vi "Update Pin Map.vi"(8 "error in":errorcluster, 11 "Pin Map Path":string) -> (0 "error out":errorcluster, 3 "Pin Map Id Out":string)   [LabVIEW 2020, in "NIDCPowerSourceDCVoltage.lvlib"]
uses:
  NIDCPowerSourceDCVoltage.lvlib
  <vilib>/MeasurementLink/MeasurementLink Discovery Client/RPC Messages/ni_measurementlink_discovery_v1_ResolveServiceRequest.ctl
  <vilib>/MeasurementLink/MeasurementLink Pin Map Client/RPC Messages/ni_measurementlink_pinmap_v1_UpdatePinMapFromXmlRequest.ctl
  <vilib>/MeasurementLink/MeasurementLink Measurement Server/MeasurementLink Measurement Server.lvlib
  <vilib>/MeasurementLink/MeasurementLink Discovery Client/MeasurementLink Discovery Client.lvlib
  <vilib>/MeasurementLink/MeasurementLink Pin Map Client/MeasurementLink Pin Map Client.lvlib
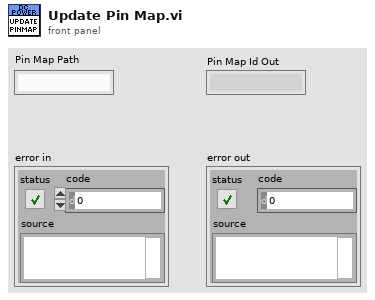
[diagram p1: front panel]
types:
  T1 = typedef "MeasurementLink Pin Map Client.lvlib/ni_measurementlink_pinmap_v1_UpdatePinMapFromXmlRequest.ctl" = cluster{"pin_map_id":string, "pin_map_xml":string}
  T2 = typedef "MeasurementLink Discovery Client.lvlib/ni_measurementlink_discovery_v1_ResolveServiceRequest.ctl" = cluster{"provided_interface":string, "service_class":string}
  T3 = typedef "grpc-lvsupport-release.lvlib/grpcId.ctl" = u64
  T4 = typedef "MeasurementLink Discovery Client.lvlib/ni_measurementlink_discovery_v1_ServiceLocation.ctl" = cluster{"location":string, "insecure_port":string, "ssl_authenticated_port":string}
  T5 = typedef "MeasurementLink Pin Map Client.lvlib/ni_measurementlink_pinmap_v1_PinMap.ctl" = cluster{"pin_map_id":string}
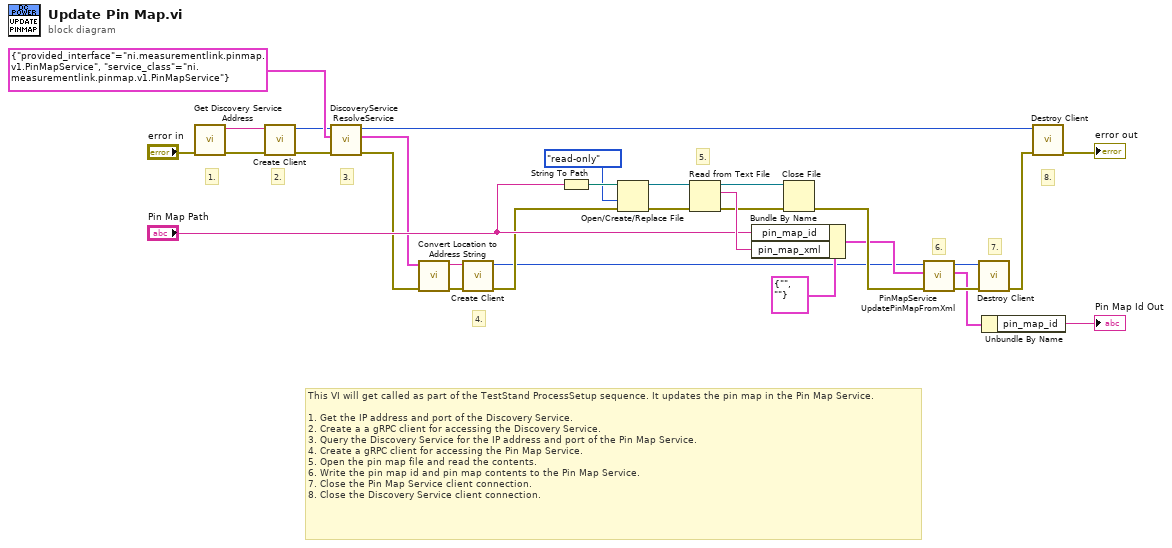
[diagram p0: block diagram]
diagram:
  # "8."
  # "7."
  # "6."
  # "5."
  # "4."
  # "3."
  # "2."
  # "1."
  # "This VI will get called as part of the TestStand ProcessSetup sequence. It updates the pin map in the Pin Map Service. \n\n1. Get the IP address and port of the Discovery Service.\n2. Create a a gRPC client for accessing the Discovery Service.\n3. Query the Discovery Service for the IP address and port of the Pin Map Service.\n4. Create a gRPC client for accessing the Pin Map Service.\n5. Open the pin map file and read the contents.\n6. Write the pin map id and pin map contents to the Pin Map Service.\n7. Close the Pin Map Service client connection.\n8. Close the Discovery Service client connection."
  n1 = call <vilib>:"Get Discovery Service Address.vi"("error in"="error in") -> ("error out"=w29:errorcluster, "address"=w28:string)  [unwired: 9 in]
  n2 = call <vilib>:"Create Client.vi"("error in"=w29, "address"=w28) -> ("error out"=w16:errorcluster, "gRPC ID Out"=w26:T3)  [unwired: 8 in]
  n3 = call <vilib>:"DiscoveryService ResolveService.vi"("error in"=w16, "Request Data"=T2 {"provided_interface"="ni.measurementlink.pinmap.v1.PinMapService", "service_class"="ni.measurementlink.pinmap.v1.PinMapService"}, "gRPC ID"=w26) -> ("error out"=w15:errorcluster, "Response Data"=w4:T4, "gRPC ID out"=w5:T3)  [unwired: 6 in]
  n4 = call "Convert Location to Address String.vi"("Response Data"=w4) -> ("String"=w3:string)  [unwired: 10 in]
  n5 = call <vilib>:"Create Client.vi"("error in"=w15, "address"=w3) -> ("error out"=w14:errorcluster, "gRPC ID Out"=w10:T3)  [unwired: 8 in]
  n6 = String To Path(string="Pin Map Path") -> (path=w24:path)
  n7 = Open/Create/Replace File(file path (use dialog)=w24, error in=w14, access (0:read/write)=enum16{"read/write", "read-only", "write-only"}."read-only") -> (refnum out=w21:refnum<file>, error out=w22:errorcluster)  [unwired: 3 in, 1 out]
  n8 = Read from Text File(file (use dialog)=w21, error in=w22) -> (refnum out=w17:refnum<file>, text=w20:string, error out=w18:errorcluster)  [unwired: 2 in, 1 out]
  n9 = Bundle By Name(cluster=T1 {"pin_map_id"="", "pin_map_xml"=""} ("Request Data"), "pin_map_id"="Pin Map Path", "pin_map_xml"=w20) -> (w11:T1)
  n10 = Close File(refnum=w17, error in=w18) -> (error out=w13:errorcluster)  [unwired: 1 out]
  n11 = call <vilib>:"PinMapService UpdatePinMapFromXml.vi"("error in"=w13, "Request Data"=w11, "gRPC ID"=w10) -> ("error out"=w9:errorcluster, "Response Data"=w2:T5, "gRPC ID out"=w8:T3)  [unwired: 6 in]
  n12 = call <vilib>:"Destroy Client.vi"("error in"=w9, "gRPC ID"=w8) -> ("error out"=w7:errorcluster)  [unwired: 9 in]
  n13 = Unbundle By Name(w2) -> ("pin_map_id"=→"Pin Map Id Out":string)
  n14 = call <vilib>:"Destroy Client.vi"("error in"=w7, "gRPC ID"=w5) -> ("error out"=→"error out":errorcluster)  [unwired: 9 in]
